vi "FTW-Actor-Connection-Add.vi"(0 "FTW-ActorExtended In":refnum<class "FTW-ActorInstance.lvclass">, 5 "Name":string, 7 "Inbox Address":string, 11 "error in":errorcluster) -> (4 "FTW-ActorExtended Out":refnum<class "FTW-ActorInstance.lvclass">, 15 "error out":errorcluster)   [LabVIEW 2015, in "FTW-ActorInstance.lvclass"]
uses:
  FTW-ActorInstance.lvclass
  Connector/FTW-ActorConnector.lvclass
  FTW-ActorInstance.lvclass/FTW-ActorInstance.ctl
  Ether/FTW-Ether.lvclass
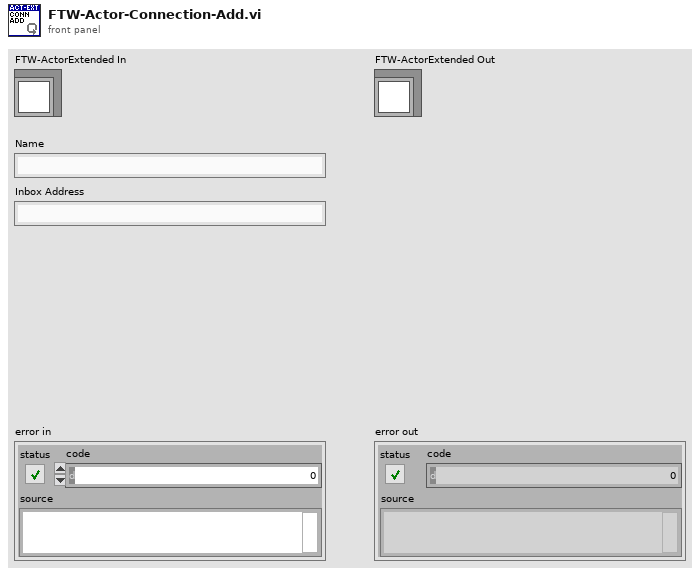
[diagram p1: front panel]
types:
  T1 = cluster{"Name":string, "Fetched Address":string, "FTW Actor Connector":refnum<class "FTW-ActorConnector.lvclass">, bool}
  T2 = cluster{"Name":string, "URI":string, "Connector":refnum<class "FTW-ActorConnector.lvclass">, "Child":bool}[]
  T3 = cluster{"Name":string, "Fetched Address":string, "FTW Actor Connector":refnum<class "FTW-ActorConnector.lvclass">, "Child":bool}[]
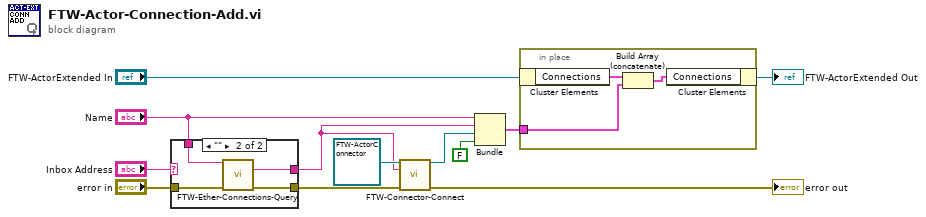
[diagram p0: block diagram]
diagram:
  n1 = case shown="\"\"" "Inbox Address" {
    selector: "Inbox Address" -> [w14 _]
    tunnel: "error in" -> [w13 w18]
    tunnel: [w13 w17] -> w7
    tunnel: "Name" -> [_ w16]
    tunnel: [w14 w15] -> w6
    frame Default {
    }
    frame "" {
      n2 = call "FTW-Ether-Connections-Query.vi"("Connection"=w16, "error in"=w18) -> ("Fetched Address"=w15:string, "error out"=w17:errorcluster)  [unwired: 12 in]
    }
  }
  n3 = call-dynamic "FTW-Connector-Connect.vi"("FTW Actor Connector Type"=refnum<class "FTW-ActorConnector.lvclass"> refnum, "Instance Inbox Address"=w6, "error in"=w7) -> ("FTW Actor Connector"=w9:refnum<class "FTW-ActorConnector.lvclass">, "error out"=→"error out":errorcluster)  [unwired: 11 in]
  n4 = Bundle("Name"="Name", "Fetched Address"=w6, "FTW Actor Connector"=w9, FALSE) -> (w1:T1)  [unwired: 1 in]
  n5 = in-place {
    in-place-border: w1 -> [w19]
    n6 = in-place-cluster #1("FTW-ActorExtended In") -> ("Connections"=w21:T2)
    n7 = Build Array (concatenate)(w21, w19) -> (w20:T3)
    n8 = in-place-cluster #1("Connections"=w20) -> (→"FTW-ActorExtended Out":refnum<class "FTW-ActorInstance.lvclass">)
  }
